vi "Divide Rational Polynomials (CDB).vi"(4 "threshold type":T1 items=["Absolute Value", "Relative Value"], 6 "threshold":dbl, 8 "Denominator 2":cdb[](array[numeric]) format="%#.2g", 9 "Numerator 2":cdb[](array[numeric]) format="%#.2g", 10 "Denominator 1":cdb[](array[numeric]) format="%#.2g", 11 "Numerator 1":cdb[](array[numeric]) format="%#.2g") -> (0 "error":i32, 2 "Denominator Out":cdb[](array[numeric]) format="%#.2g", 3 "Numerator Out":cdb[](array[numeric]) format="%#.2g")   [LabVIEW 2020, in "NI_AALPro.lvlib"]
doc: "Divides rational polynomial G1 by rational polynomial G2. The data types you wire to the <B>Numerator 1</B>, <B>Denominator 1</B>, <B>Numerator 2</B>, and <B>Denominator 2</B> inputs determine the polymorphic instance to use."
uses:
  NI_AALPro.lvlib
  Remove Zero Threshold Type.ctl
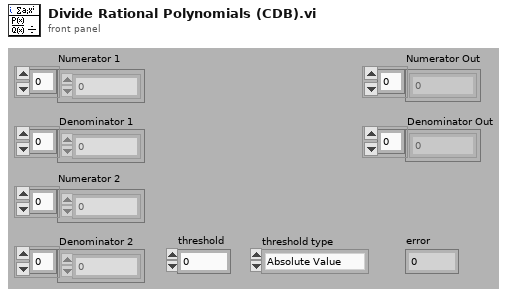
[diagram p1: front panel]
types:
  T1 = typedef "NI_AALPro.lvlib/Remove Zero Threshold Type.ctl" = u16
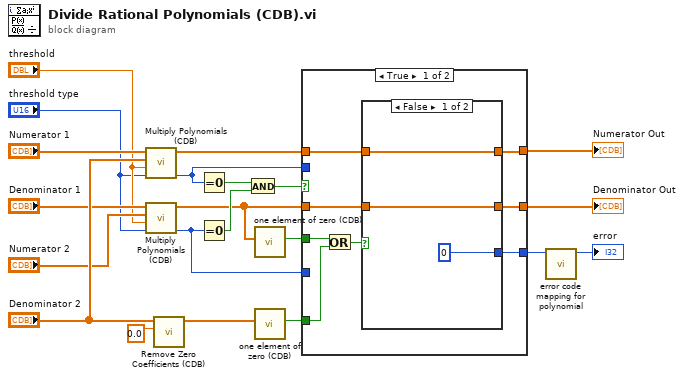
[diagram p0: block diagram]
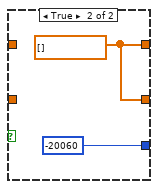
[diagram p2: hidden frame]
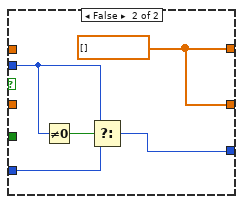
[diagram p3: hidden frame]
diagram:
  n1 = call "Multiply Polynomials (CDB).vi"("threshold type"="threshold type", "threshold"="threshold", "Q(x)"="Denominator 2", "P(x)"="Numerator 1") -> ("error"=w9:i32, "P(x)*Q(x)"=w6:cdb[])  [unwired: 6 in]
  n2 = call "Multiply Polynomials (CDB).vi"("threshold type"="threshold type", "threshold"="threshold", "Q(x)"="Numerator 2", "P(x)"="Denominator 1") -> ("error"=w11:i32, "P(x)*Q(x)"=w1:cdb[])  [unwired: 6 in]
  n3 = call "Remove Zero Coefficients (CDB).vi"("threshold"=0.0, "P(x) In"="Denominator 2") -> ("P(x) Out"=w18:cdb[])  [unwired: 7 in, 2 out]
  n4 = Equal To 0?(x=w9) -> (x = 0?=w13:bool)
  n5 = Equal To 0?(x=w11) -> (x = 0?=w10:bool)
  n6 = And(x=w13, y=w10) -> (x .and. y?=w12:bool)
  n7 = call "one element of zero (CDB).vi"("Array in"=w1) -> ("equal [0]?"=w17:bool)  [unwired: 10 in]
  n8 = call "one element of zero (CDB).vi"("Array in"=w18) -> ("equal [0]?"=w16:bool)  [unwired: 10 in]
  n9 = case shown="True" w12 {
    tunnel: w6 -> [w29 _]
    tunnel: w1 -> [w28 _]
    tunnel: [w27 w39] -> w21
    tunnel: [w26 w39] -> w20
    tunnel: [w25 w35] -> w15
    tunnel: w17 -> [w23 _]
    tunnel: w16 -> [w22 _]
    tunnel: w11 -> [_ w36]
    tunnel: w9 -> [_ w37]
    frame True {
      n10 = Or(x=w23, y=w22) -> (x .or. y?=w24:bool)
      n11 = case shown="False" w24 {
        tunnel: w29 -> [w32 _]
        tunnel: w28 -> [w31 _]
        tunnel: [w32 w33] -> w27
        tunnel: [w31 w33] -> w26
        tunnel: [0 -20060 ("divide by zero")] -> w25
        frame False {
        }
        frame True {
          w33 = cdb[] [] ("CDB")
        }
      }
    }
    frame False {
      w39 = cdb[] [] ("CDB")
      n12 = Not Equal To 0?(x=w37) -> (x != 0?=w38:bool)
      n13 = Select(t=w37, s=w38, f=w36) -> (s? t:f=w35:i32)
    }
  }
  "Numerator Out" <- w21
  "Denominator Out" <- w20
  n14 = call "error code mapping for polynomial.vi"("error in"=w15) -> ("error out"=→"error":i32)  [unwired: 10 in]
